vi "pharosGenerateTriggers.vi"() -> (0 "triggers":u8[](array[numeric]))   [LabVIEW 2017]
uses:
  globalUtilities.vi
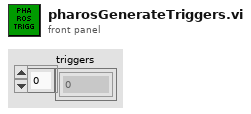
[diagram p1: front panel]
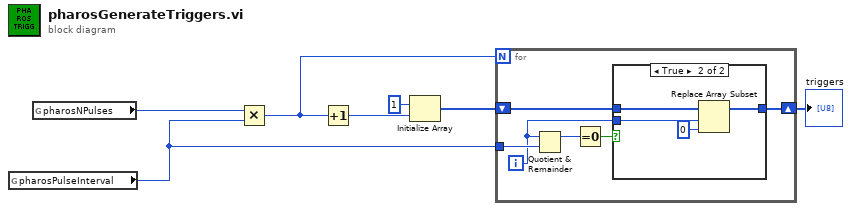
[diagram p0: block diagram]
diagram:
  n1 = global read "globalUtilities.vi" "pharosPulseInterval"() -> (w1:i32)
  n2 = global read "globalUtilities.vi" "pharosNPulses"() -> (w2:i32)
  n3 = Multiply(x=w2, y=w1) -> (x*y=w5:i32)
  n4 = Increment(x=w5) -> (x+1=w7:i32)
  n5 = Initialize Array(u8 1 ("element"), w7) -> (w4:u8[])
  n6 = for {
    N: w5 -> [_]
    tunnel: w1 -> [w12]
    shift-right: [w8] -> w3
    shift-left: w4 -> [w13]
    i -> [w9]
    n7 = Quotient & Remainder(x=w9, y=w12) -> (x-y*floor(x/y)=w11:i32)  [unwired: 1 out]
    n8 = Equal To 0?(x=w11) -> (x = 0?=w10:bool)
    n9 = case shown="True" w10 {
      tunnel: w13 -> [w14 w18]
      tunnel: w9 -> [_ w17]
      tunnel: [w14 w15] -> w8
      frame False {
      }
      frame True {
        n10 = Replace Array Subset(array=w18, new element=u8 0 ("new element/subarray"), index=w17) -> (w15:u8[])
      }
    }
  }
  "triggers" <- w3
